vi "Create RDB Objects.vi"(8 "error in":errorcluster, 10 "Channel Refs in":T2[](array[typedef]) format="%.0x", 11 "PlayerID":u8) -> (0 "error out":errorcluster, 3 "RDB OBJs":T1[](array[typedef]))   [LabVIEW 2023, in "Vires VTD System Explorer.lvlib"]
uses:
  Vires VTD System Explorer.lvlib
  <vilib>/NI VeriStand/Custom Device API/Custom Device Item Ref.ctl
  RDB/RDB Player Object.ctl
  <vilib>/NI VeriStand/Custom Device API/Get Item Property (Variant).vi
  <vilib>/NI VeriStand/Custom Device API/Custom Device API.lvlib
  RDB/RDB.lvlib
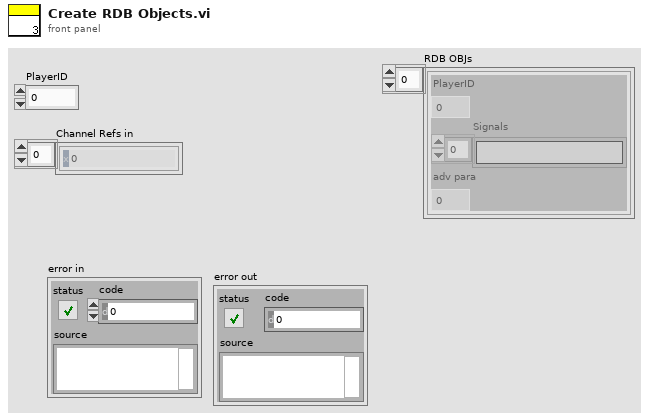
[diagram p1: front panel]
types:
  T1 = typedef "RDB.lvlib/RDB Player Object.ctl" = cluster{"PlayerID":i32, "Signals":string[], "adv para":i32}
  T2 = typedef "Custom Device API.lvlib/Custom Device Item Ref.ctl" = u64
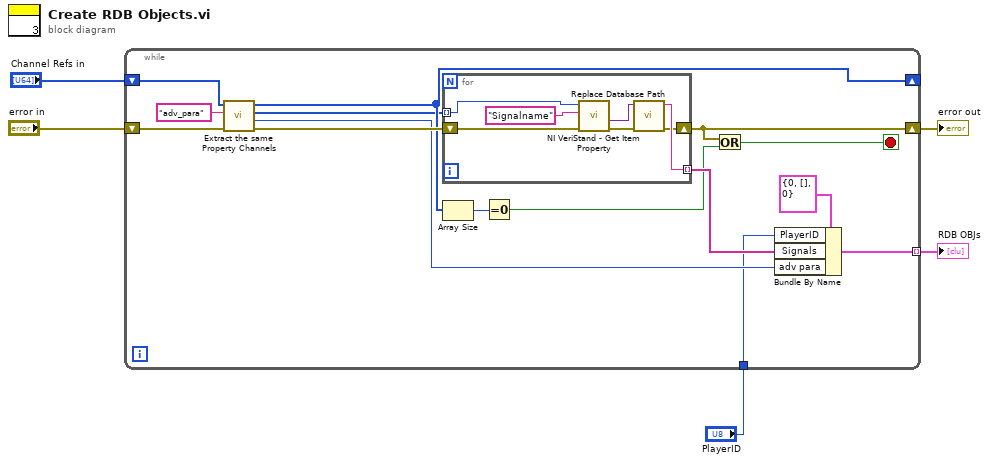
[diagram p0: block diagram]
diagram:
  n1 = while {
    shift-right: [w12] -> w4
    shift-left: "error in" -> [w16]
    tunnel: [w15] -> w3 mode=indexing
    shift-right: [w9] -> _
    shift-left: "Channel Refs in" -> [w18]
    tunnel: "PlayerID" -> [w6]
    stop <- w7 stop-if-true
    n2 = call "Extract the same Property Channels.vi"("error in (no error)"=w16, "Property Name"="adv_para", "Channel Refs in"=w18) -> ("error out"=w17:errorcluster, "Property Value"=w11:u8, "Extracted the same pkid Channel Refs"=w8:T2[], "Channel Refs Remaining"=w9:T2[])  [unwired: 5 in]
    n3 = for {
      shift-right: [w22] -> w12
      shift-left: w17 -> [w24]
      tunnel: [w23] -> w19 mode=indexing
      tunnel: w8 -> [w21] mode=indexing
      n4 = call-poly <vilib>:"NI VeriStand - Get Item Property.vi"("error in (no error)"=w24, "Property Name"="Signalname", "Item Ref in"=w21) -> ("error out"=w26:errorcluster, "Value"=w27:variant)  [unwired: 5 in, 2 out]
      n5 = call "Replace Database Path.vi"("error in (no error)"=w26, "Value"=w27) -> ("error out"=w22:errorcluster, "Property Name"=w23:string)  [unwired: 8 in]
    }
    n6 = Array Size(array=w9) -> (size(s)=w13:i32)
    n7 = Equal To 0?(x=w13) -> (x = 0?=w14:bool)
    n8 = Or(x=w12, y=w14) -> (x .or. y?=w7:bool)
    n9 = Bundle By Name(cluster=T1 {"PlayerID"=0, "Signals"=[], "adv para"=0} ("RDB Player Objects"), "PlayerID"=w6, "Signals"=w19, "adv para"=w11) -> (w15:T1)
  }
  "error out" <- w4
  "RDB OBJs" <- w3
